vi "set filter (waveform).vi"(8 "error in (no error)":errorcluster, 9 "Include Only Visible?":bool, 10 "Type":enum16{"All", "DBL", "CDB"}(ring), 11 "abstract-tree in":refnum<class "abstract-tree.lvclass">) -> (0 "error out":errorcluster, 3 "abstract-tree out":refnum<class "abstract-tree.lvclass">)   [LabVIEW 2017]
uses:
  abstract-tree.lvclass
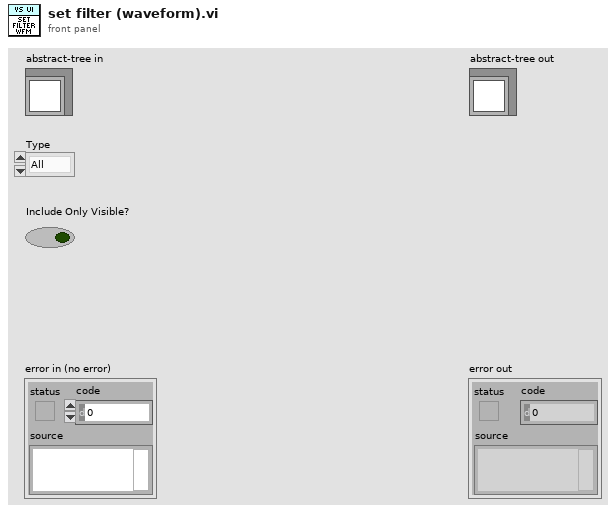
[diagram p1: front panel]
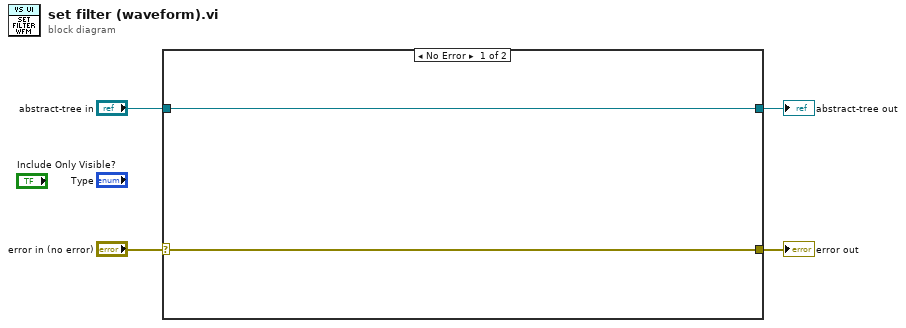
[diagram p0: block diagram]
diagram:
  n1 = case shown="No Error" "error in (no error)" {
    selector: "error in (no error)" -> [w6 w8]
    tunnel: [w6 w8] -> w3
    tunnel: [w5 w7] -> w1
    tunnel: "abstract-tree in" -> [w5 w7]
    frame No Error {
    }
    frame Error {
    }
  }
  "error out" <- w3
  "abstract-tree out" <- w1
